vi "Read UID.vi"(9 "GObject in":refnum<class "GObject.lvclass">) -> (3 "GObject out":refnum<class "GObject.lvclass">, 4 "UID":i32)   [LabVIEW 2014, in "GObject.lvclass"]
uses:
  GObject.lvclass
  GObject.lvclass/GObject.ctl
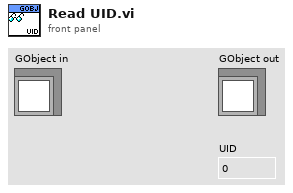
[diagram p1: front panel]
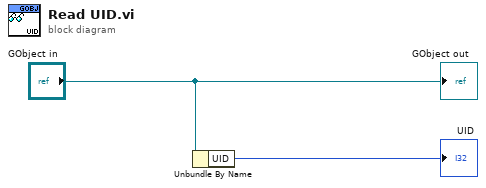
[diagram p0: block diagram]
diagram:
  n1 = Unbundle By Name("GObject in") -> ("UID"=→"UID":i32)
  "GObject out" <- "GObject in"
